vi "Send Toggle Display.vi"(8 "error in":errorcluster, 10 "Show":bool, 11 "Fault Handler in":refnum<class "Fault Handler.lvclass">) -> (0 "error out":errorcluster, 3 "Fault Handler out":refnum<class "Fault Handler.lvclass">)   [LabVIEW 2023, in "Fault Handler.lvlib" / "Fault Handler.lvclass"]
doc: "This routine transmits the toggle display command implemented at the <b>Main UI</b> level."
uses:
  Library/Fault Handler.lvclass
  C:/Users/Public/Documents/Development/builds/Engine/Engine.lvlibp/Project/Engine.lvclass
  C:/Users/Public/Documents/Development/builds/Engine/Actor Framework.lvlibp/1abvi3w/vi.lib/ActorFramework/Actor/Actor.lvclass
  builds/Engine/Engine.lvlibp/Accessors/Read Caller Q.vi
  builds/Engine/Actor Framework.lvlibp/1abvi3w/vi.lib/ActorFramework/Actor/Read Actor Label.vi
  builds/Engine/Actor Framework.lvlibp/1abvi3w/vi.lib/ActorFramework/Message Enqueuer/Message Enqueuer.lvclass
  builds/Engine/Engine.lvlibp/Engine Messages/Toggle Component Display Msg/Toggle Component Display Msg.lvclass
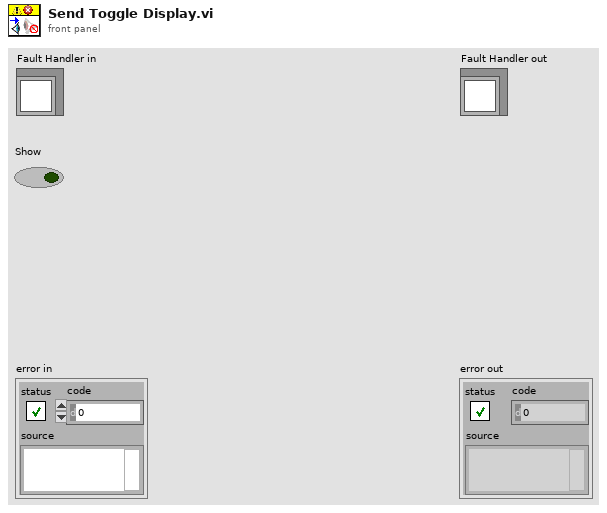
[diagram p1: front panel]
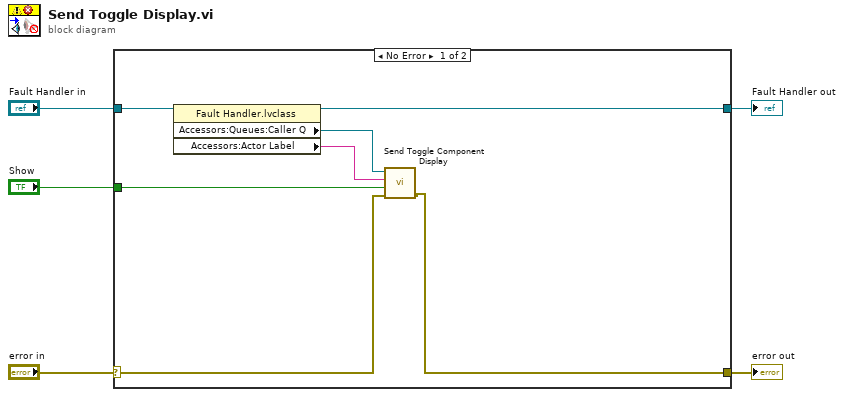
[diagram p0: block diagram]
diagram:
  n1 = case shown="No Error" "error in" {
    selector: "error in" -> [w10 w14]
    tunnel: [w9 w14] -> w4
    tunnel: [w11 w13] -> w2
    tunnel: "Fault Handler in" -> [w12 w13]
    tunnel: "Show" -> [w6 _]
    frame No Error {
      n2 = property class="Fault Handler.lvclass"(reference=w12) -> (reference out=w11:refnum<class "Fault Handler.lvclass">, "Accessors:Queues:Caller Q"=w8:refnum<class "Message Enqueuer.lvclass">, "Accessors:Actor Label"=w7:string)  [unwired: 1 in, 1 out]
      n3 = call "Send Toggle Component Display.vi"("error in (no error)"=w10, "Show"=w6, "Identifier"=w7, "Message Enqueuer"=w8) -> ("error out"=w9:errorcluster)  [unwired: 6 in, 1 out]
    }
    frame Error {
    }
  }
  "error out" <- w4
  "Fault Handler out" <- w2
